vi "Autonomous Shooting.vi"() -> ()   [LabVIEW 2012]
panel:
  in  "Autonomous Shooting":bool
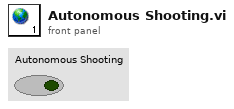
[diagram p1: front panel]
diagram:
